vi "Print Reset.vi"(8 "error in (no error)":errorcluster, 11 "Feeder Actor.lvlib:Feeder.lvclass":refnum<class "Feeder.lvclass">) -> (0 "error out":errorcluster, 3 "Feeder Actor.lvlib:Feeder.lvclass 2":refnum<class "Feeder.lvclass">)   [LabVIEW 2018, in "Feeder Actor.lvlib" / "Feeder.lvclass"]
uses:
  Feeder.lvclass
  Feeder.lvclass/Feeder.ctl
  Solenoid Messages/Set Solonoid Msg/Set Solonoid Msg.lvclass/Set Solonoid Msg.ctl
  <vilib>/ActorFramework/Message Enqueuer/Message Enqueuer.lvclass/Message Enqueuer.ctl
  <vilib>/ActorFramework/Message Enqueuer/Enqueue.vi
  Solenoid Messages/Set Solonoid Msg/Set Solonoid Msg.lvclass
  C:/Program Files/National Instruments/LabVIEW 2018/vi.lib/ActorFramework/Message/Message.lvclass
  <vilib>/ActorFramework/Message Priority Queue/Priority Enqueue.vi
  Screw Messages/Screw Print Msg/Screw Print Msg.lvclass
  Mixer Messages/Mixer Print Msg/Mixer Print Msg.lvclass
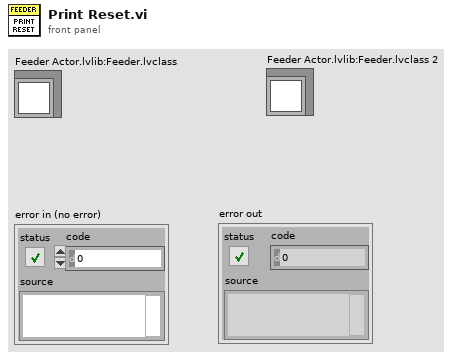
[diagram p1: front panel]
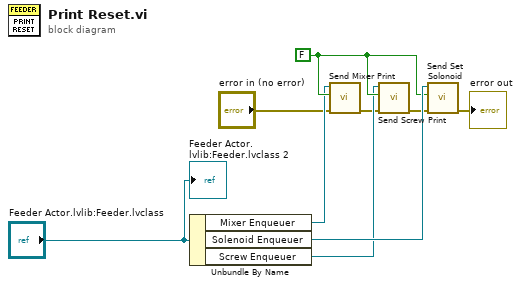
[diagram p0: block diagram]
diagram:
  w6 = FALSE ("State")
  n1 = Unbundle By Name("Feeder Actor.lvlib:Feeder.lvclass") -> ("Mixer Enqueuer"=w5:refnum<class "Message Enqueuer.lvclass">, "Solenoid Enqueuer"=w8:refnum<class "Message Enqueuer.lvclass">, "Screw Enqueuer"=w4:refnum<class "Message Enqueuer.lvclass">)
  n2 = call "Send Mixer Print.vi"("error in (no error)"="error in (no error)", "On?"=w6, "Message Enqueuer in"=w5) -> ("error out"=w2:errorcluster)  [unwired: 7 in, 1 out]
  n3 = call "Send Screw Print.vi"("error in (no error)"=w2, "On?"=w6, "Message Enqueuer in"=w4) -> ("error out"=w3:errorcluster)  [unwired: 7 in, 1 out]
  n4 = call "Send Set Solonoid.vi"("error in (no error)"=w3, "State"=w6, "Message Enqueuer in"=w8) -> ("error out"=→"error out":errorcluster)  [unwired: 7 in, 1 out]
  "Feeder Actor.lvlib:Feeder.lvclass 2" <- "Feeder Actor.lvlib:Feeder.lvclass"
